vi "CMI ckd2 Panel.vi"(8 "error in":errorcluster, 11 "session":T1) -> (0 "error out":errorcluster, 3 "session out":T1)   [LabVIEW 2020, in "AWG.lvlib"]
doc: "CMI clock divider v2 configuration panel."
uses:
  AWG.lvlib
  CMI ckd2 Session.ctl
  CMI ckd2 Source Mode.ctl
panel:
  in  "btn ok":bool
  in  "Use manual reference frequency entry":bool
  in  "Manual reference clock [Hz]":dbl format="%#_8p"
  in  "Clock source":T2
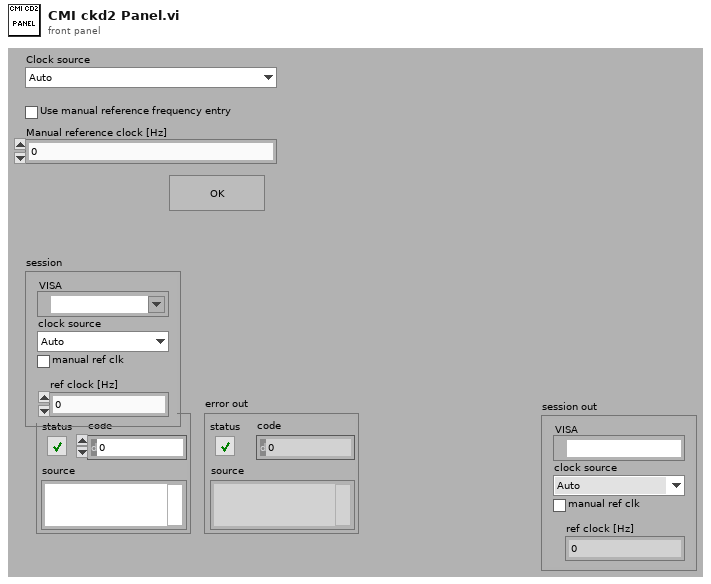
[diagram p1: front panel]
types:
  T1 = typedef "AWG.lvlib/CMI ckd2 Session.ctl" = cluster{"VISA":refnum<visa-resource-name>, "clock source":T2, "manual ref clk":bool, "ref clock [Hz]":dbl}
  T2 = typedef "AWG.lvlib/CMI ckd2 Source Mode.ctl" = enum16{"Auto", "LF clock", "HF clock", "Internal"}
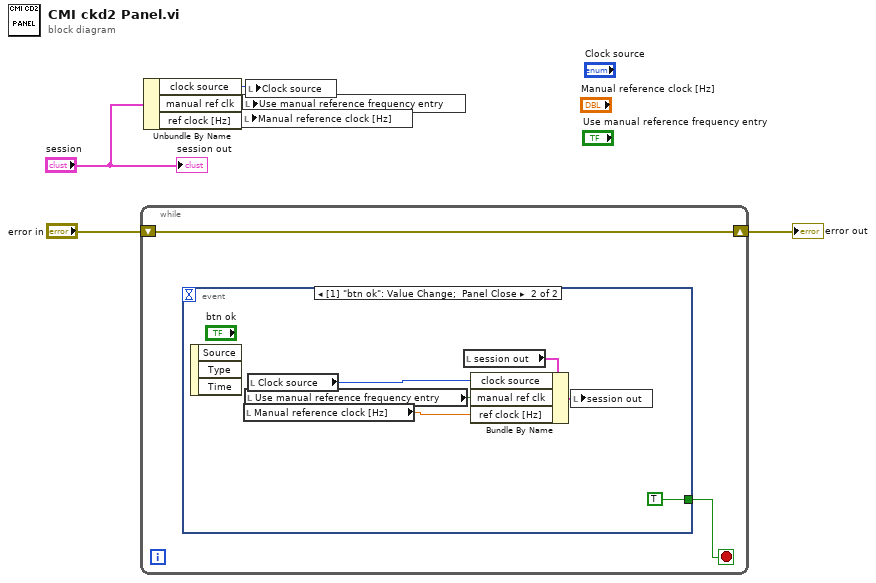
[diagram p0: block diagram]
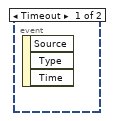
[diagram p2: hidden frame]
diagram:
  n1 = while {
    shift-right: [w7] -> w3
    shift-left: "error in" -> [w7]
    stop <- w8 stop-if-true
    n2 = event shown="[1] \"btn ok\": Value Change;  Panel Close" {
      selector: _ -> [_ _]
      dyn-events: _ -> [_ _]
      timeout: _ -> [_ _]
      tunnel: [_ TRUE] -> w8
      event Timeout {
        n3 = event-data() -> ()  [unwired: 1 in, 3 out]
      }
      event "btn ok": Value Change; Panel Close {
        n4 = event-data() -> ()  [unwired: 1 in, 3 out]
        n5 = local read "Manual reference clock [Hz]"() -> (w10:dbl)
        n6 = local read "Use manual reference frequency entry"() -> (w11:bool)
        n7 = local read "Clock source"() -> (w12:T2)
        n8 = local read "session out"() -> (w13:T1)
        n9 = Bundle By Name(cluster=w13, "clock source"=w12, "manual ref clk"=w11, "ref clock [Hz]"=w10) -> (w9:T1)
        n10 = local write "session out"(w9) -> ()
      }
    }
  }
  "error out" <- w3
  n11 = Unbundle By Name("session") -> ("clock source"=w6:T2, "manual ref clk"=w5:bool, "ref clock [Hz]"=w4:dbl)
  n12 = local write "Manual reference clock [Hz]"(w4) -> ()
  n13 = local write "Use manual reference frequency entry"(w5) -> ()
  n14 = local write "Clock source"(w6) -> ()
  "session out" <- "session"
